vi "SamplekFifoSetup.vi"() -> ()   [LabVIEW 2010, in "kevLib2011.lvlib"]
uses:
  kevLib2011.lvlib
panel:
  out "fifo full counter":u16
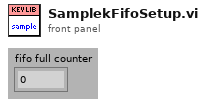
[diagram p1: front panel]
types:
  T1 = cluster{"Fifo Size":u32, "FileRefnum":refnum<file>, "FifoRefnum":refnum<k33>, "Fifo Time Out (ms)":i32, "MaxNumFileWrite":i32, "Force Num Array":i32}
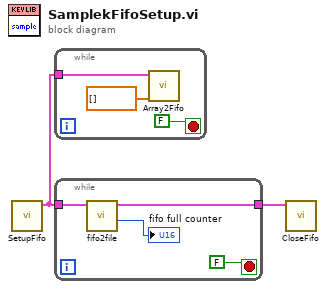
[diagram p0: block diagram]
diagram:
  n1 = call "SetupFifo.vi"() -> ("Data Logging Param"=w2:T1)  [unwired: 11 in]
  n2 = while {
    tunnel: w2 -> [w5]
    stop <- FALSE stop-if-true
    n3 = call "Array2Fifo.vi"("Input Array"=dbl[] [], "DataLoggingParam"=w5) -> ()  [unwired: 10 in]
  }
  n4 = while {
    tunnel: w2 -> [w9]
    tunnel: [w8] -> w1
    stop <- FALSE stop-if-true
    n5 = call "fifo2file.vi"("DataLoggingParam"=w9) -> ("fifo full counter"=→"fifo full counter":u16, "DataLoggingParam 2"=w8:T1)  [unwired: 9 in]
  }
  n6 = call "CloseFifo.vi"("DataLoggingParam"=w1) -> ()  [unwired: 11 in]
